vi "mod_ResamplingFilter.vi"(0 "interpolation factor in":i32=128, 5 "effective filter length":i32=8, 12 "legacy filter?":bool) -> (4 "filerData[]":dbl[](array[numeric]), 6 "interpolation factor":i32=128, 8 "effective filter length":i32=16)   [LabVIEW 2020, in "niAMT.lvlib"]
uses:
  <vilib>/addons/Modulation/niAMT.lvlib
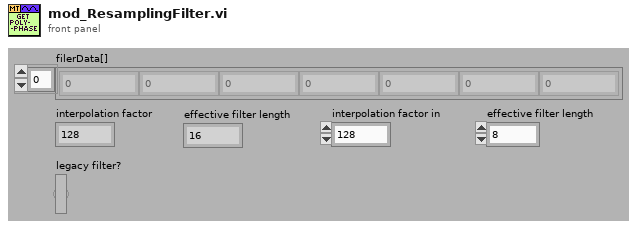
[diagram p1: front panel]
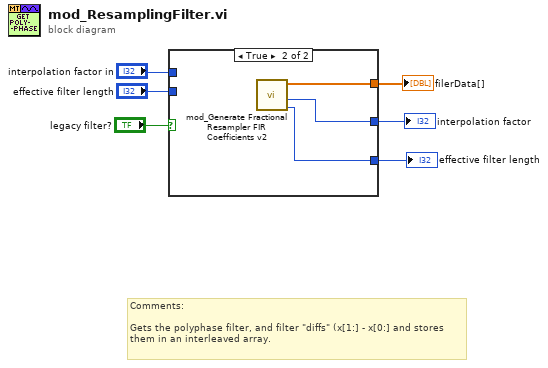
[diagram p0: block diagram]
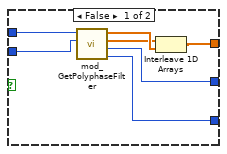
[diagram p2: hidden frame]
diagram:
  # "Comments:\n\nGets the polyphase filter, and filter \"diffs\" (x[1:] - x[0:] and stores\nthem in an interleaved array."
  n1 = case shown="True" "legacy filter?" {
    tunnel: [w11 w16] -> w6
    tunnel: "interpolation factor in" -> [w10 _]
    tunnel: "effective filter length" -> [w9 _]
    tunnel: [w8 w15] -> w3
    tunnel: [w7 w14] -> w2
    frame False {
      n2 = call <vilib>:"mod_GetPolyphaseFilter.vi"("# of zero crossings"=w9, "interpolation factor in"=w10) -> ("effective filter length"=w7:i32, "interpolation factor"=w8:i32, "differencesBetweenCoeffs[]"=w12:dbl[], "scaledFilterCoefficients[]"=w13:dbl[])  [unwired: 1 in, 5 out]
      n3 = Interleave 1D Arrays(w12, w13) -> (w11:dbl[])
    }
    frame True {
      n4 = call <vilib>:"mod_Generate Fractional Resampler FIR Coefficients v2.vi"() -> ("effective filter length"=w14:i32, "interpolation factor"=w15:i32, "polyphase filter"=w16:dbl[])  [unwired: 9 out]
    }
  }
  "filerData[]" <- w6
  "interpolation factor" <- w3
  "effective filter length" <- w2
